vi "Refresh Access Codes.vi"(8 "error in":errorcluster, 9 "Refresh Token In":string, 11 "Authorization Code In":string) -> (0 "error out":errorcluster, 1 "Refresh Token Out":string, 2 "Access Token Out":string, 3 "Auth Code Out":string)   [LabVIEW 2016]
uses:
  <vilib>/httpClient/POSTBuffer.vi
  <vilib>/addons/_JKI.lib/Serialization/JSON/JKI JSON Serialization.lvlib
  <vilib>/httpClient/LabVIEWHTTPClient.lvlib
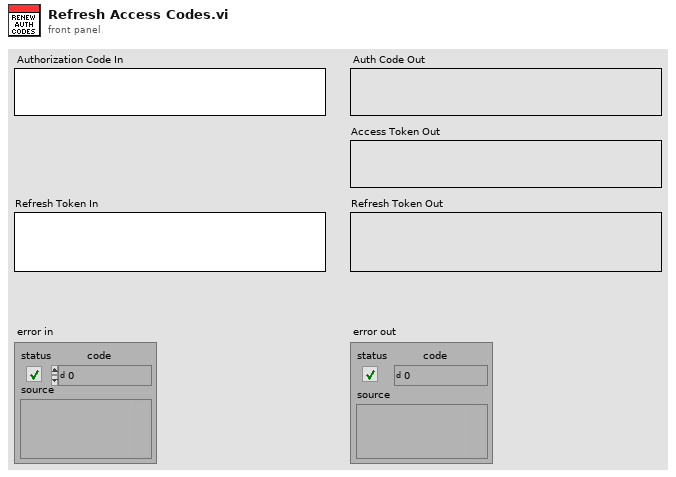
[diagram p1: front panel]
types:
  T1 = cluster{"token_type":string, "scope":string, "access_token":string, "refresh_token":string, "user_id":string, "expires_in":i32}
  T2 = typedef "LabVIEWHTTPClient.lvlib/ClientHandle.ctl" = refnum<k1>
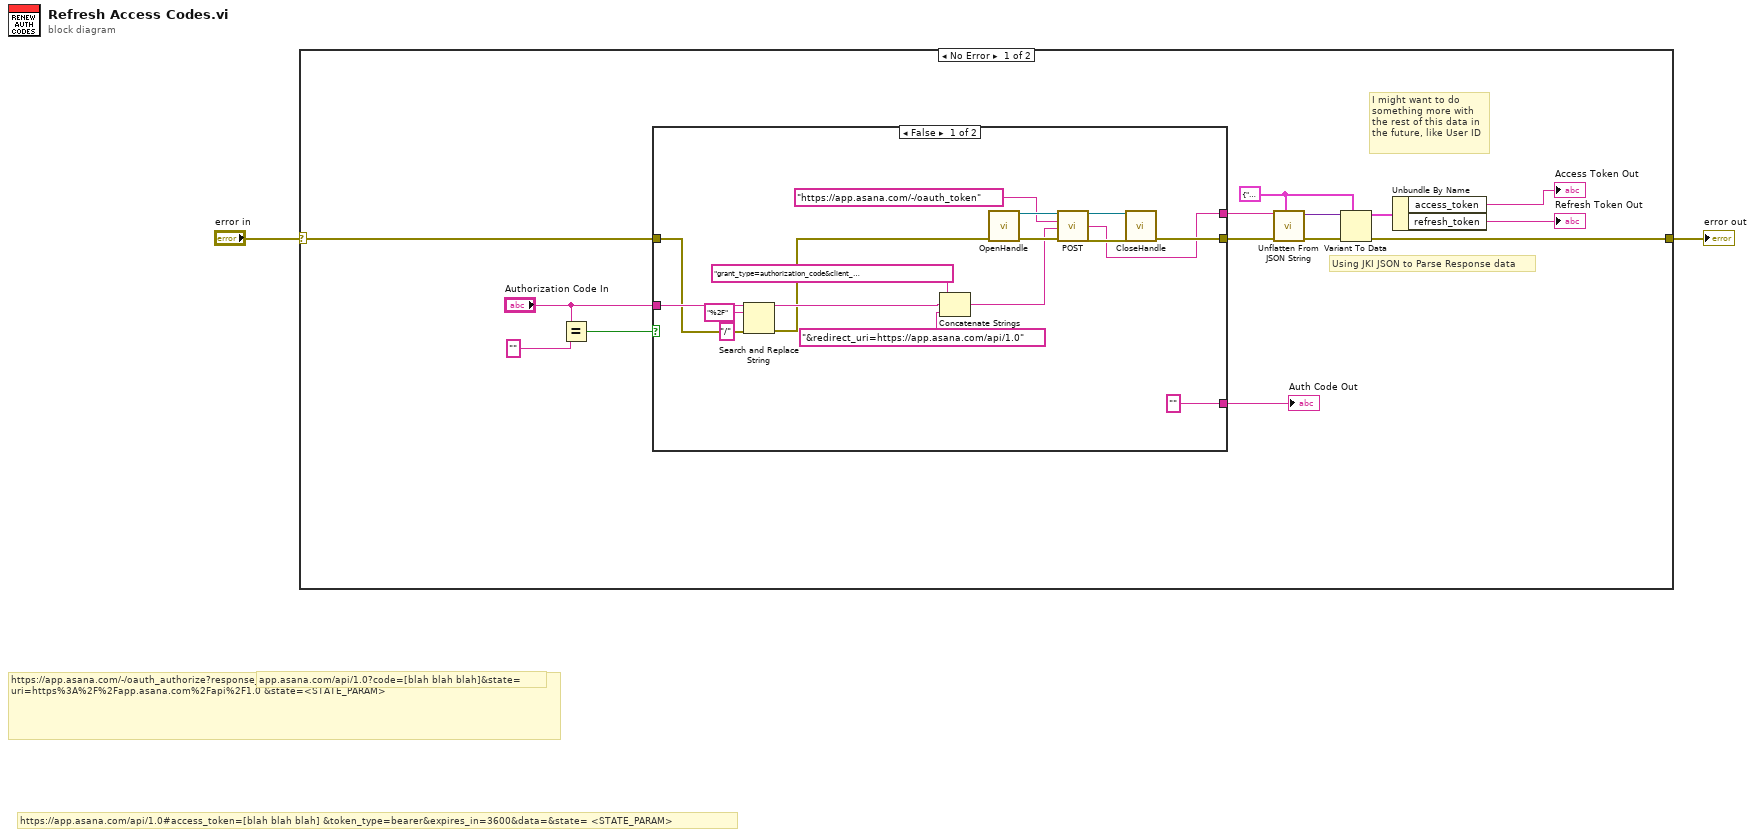
[diagram p0: block diagram]
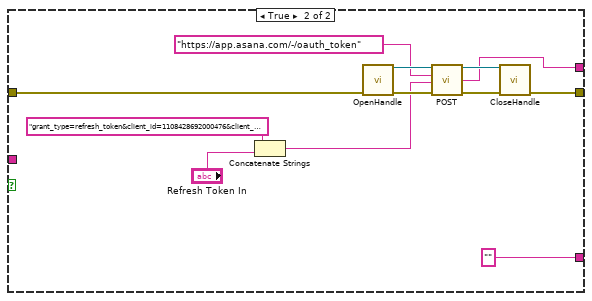
[diagram p2: hidden frame]
diagram:
  # "https://app.asana.com/api/1.0#access_token=[blah blah blah] &token_type=bearer&expires_in=3600&data=&state= <STATE_PARAM>"
  # "app.asana.com/api/1.0?code=[blah blah blah]&state="
  # "https://app.asana.com/-/oauth_authorize?response_type=code&client_id=1108428692000476&redirect_uri=https%3A%2F%2Fapp.asana.com%2Fapi%2F1.0 &state=<STATE_PARAM>"
  n1 = case shown="No Error" "error in" {
    selector: "error in" -> [w6 w46]
    tunnel: [w16 w46] -> w1
    frame No Error {
      w14 = T1 {"token_type"="", "scope"="", "access_token"="", "refresh_token"="", "user_id"="", "expires_in"=0}
      # "I might want to do something more with the rest of this data in the future, like User ID"
      # "Using JKI JSON to Parse Response data"
      n2 = Equal?(x="Authorization Code In", y="") -> (x = y?=w9:bool)
      n3 = case shown="False" w9 {
        tunnel: ["" ""] -> w7
        tunnel: w6 -> [w20 w37]
        tunnel: [w29 w34] -> w5
        tunnel: [w23 w35] -> w3
        tunnel: "Authorization Code In" -> [w22 _]
        frame False {
          n4 = Search and Replace String(input string=w22, search string="%2F", replace string="/" ("replace string (\"\")"), error in=w20) -> (result string=w21:string, error out=w19:errorcluster)  [unwired: 4 in, 2 out]
          n5 = Concatenate Strings("grant_type=authorization_code&client_id=1108428692000476&client_secret=803bdca1138fccb00921b8f346728904&code=", w21, "&redirect_uri=https://app.asana.com/api/1.0") -> (w25:string)
          n6 = call <vilib>:"OpenHandle.vi"("error in (no error)"=w19) -> ("client handle out"=w28:T2, "error out"=w31:errorcluster)  [unwired: 13 in]
          n7 = call-poly <vilib>:"POST.vi"("client handle"=w28, "url"="https://app.asana.com/-/oauth_token", "buffer"=w25, "error in (no error)"=w31) -> ("client handle out"=w27:T2, "body"=w23:string, "error out"=w30:errorcluster)  [unwired: 8 in, 1 out]
          n8 = call <vilib>:"CloseHandle.vi"("client handle"=w27, "error in (no error)"=w30) -> ("error out"=w29:errorcluster)  [unwired: 13 in]
        }
        frame True {
          n9 = Concatenate Strings("grant_type=refresh_token&client_id=1108428692000476&client_secret=803bdca1138fccb00921b8f346728904&redirect_uri=https://app.asana.com/api/1.0&refresh_token=", "Refresh Token In") -> (w36:string)
          n10 = call <vilib>:"OpenHandle.vi"("error in (no error)"=w37) -> ("client handle out"=w40:T2, "error out"=w42:errorcluster)  [unwired: 13 in]
          n11 = call-poly <vilib>:"POST.vi"("client handle"=w40, "url"="https://app.asana.com/-/oauth_token", "buffer"=w36, "error in (no error)"=w42) -> ("client handle out"=w39:T2, "body"=w35:string, "error out"=w41:errorcluster)  [unwired: 8 in, 1 out]
          n12 = call <vilib>:"CloseHandle.vi"("client handle"=w39, "error in (no error)"=w41) -> ("error out"=w34:errorcluster)  [unwired: 13 in]
        }
      }
      "Auth Code Out" <- w7
      n13 = call <vilib>:"Unflatten From JSON String.vi"("Type and Defaults"=w14, "error in (no error)"=w5, "JSON String"=w3) -> ("error out"=w15:errorcluster, "Variant"=w13:variant)  [unwired: 7 in]
      n14 = Variant To Data(error in=w15, type=w14, Variant=w13) -> (data=w12:T1, error out=w16:errorcluster)
      n15 = Unbundle By Name(w12) -> ("access_token"=→"Access Token Out":string, "refresh_token"=→"Refresh Token Out":string)
    }
    frame Error {
    }
  }
  "error out" <- w1
